vi "LVPortMakeEventStreamNameFromIDAndCategory.vi"(9 "Category":string, 11 "ID":string) -> (3 "StreamName":string)   [LabVIEW 2017]
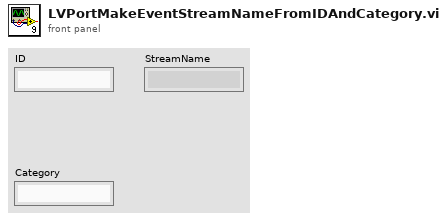
[diagram p1: front panel]
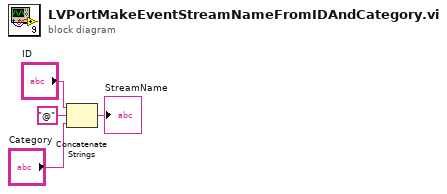
[diagram p0: block diagram]
diagram:
  n1 = Concatenate Strings("ID", "@" ("string"), "Category") -> (→"StreamName":string)
